vi "Constants.vi"() -> ()   [LabVIEW 2017, in "SLSC Switch Shared.lvlib"]
doc: "Use this Global VI to access the GUIDs assigned to the page resources of the Custom Device."
uses:
  SLSC Switch Shared.lvlib
panel:
  in  "Tab Control":enum32{"GUIDS", "Constants", "Properties"}(tab)
  in  "SLSC Switch":string="5e47c8de-3ec6-490b-8897-5526d4aea756"
  in  "Compiled.Settings":string="Compiled.Settings"
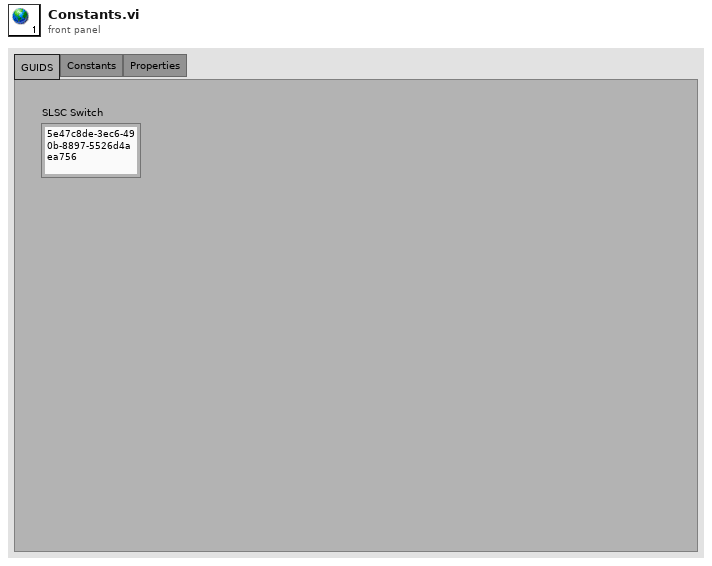
[diagram p1: front panel]
diagram:
